vi "WCA_init.vi"(8 "Cartridge band":u32=10 max=10 step=1, 10 "Node address":u16=19 format="%.0x", 11 "CAN Interface":string="CAN0") -> (0 "error out 2":errorcluster {"code" format="%.0x"}, 1 "Detected CAN Nodes.":string, 2 "Slave Node in":cluster{"Address":i16, "Serial Number":i8[]} {"Serial Number" format="%.0x"; "Address" format="%.0x"}, 3 "ObjHandle out":u32, 4 "CAN nodes found on bus.":cluster{"Address":i8, "Serial Number":i8[]}[](array[cluster]) {"Serial Number" format="%.0x"; "Address" format="%.0x"})   [LabVIEW 2017]
uses:
  WCA_Global.vi
panel:
  out "Node index Bias":i32=-1
  # "Node Address"
  # "Serial Number"
  # "Node Address"
  # "Serial Number"
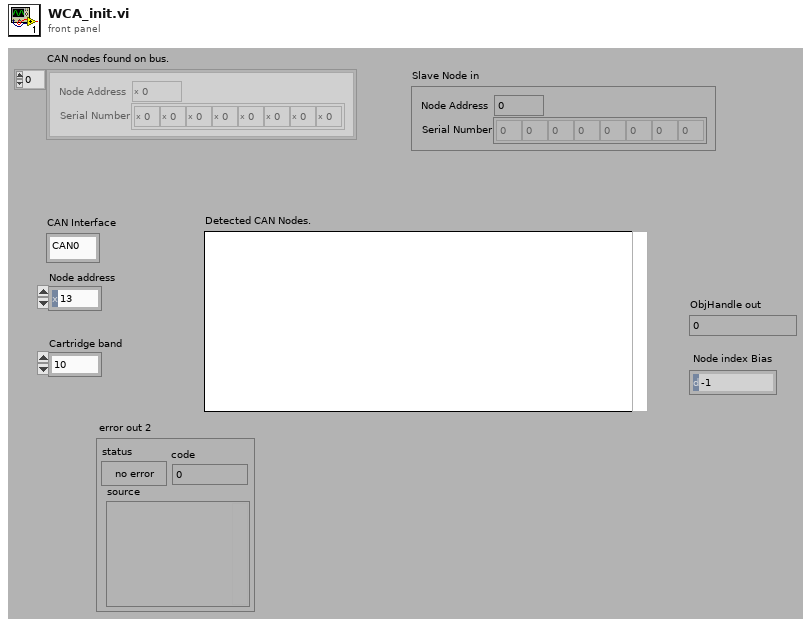
[diagram p1: front panel]
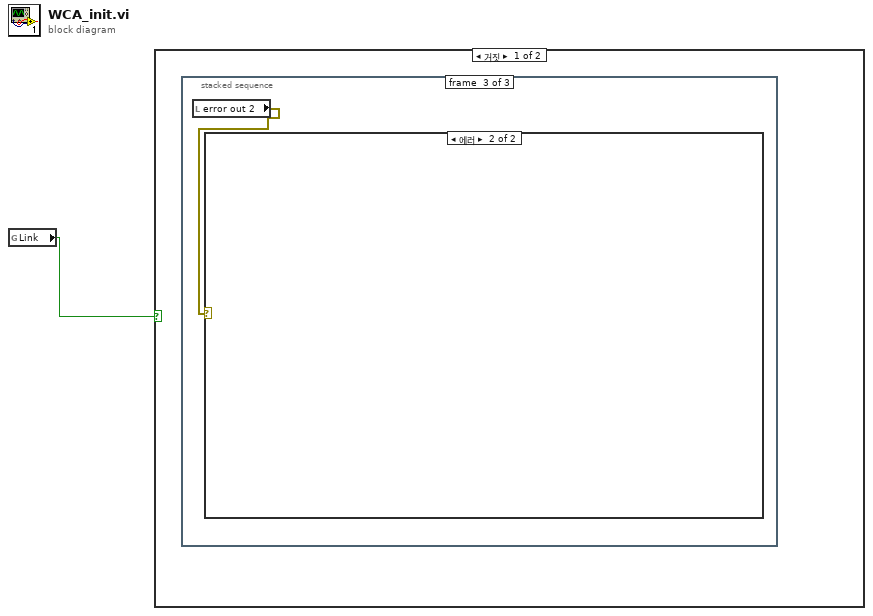
[diagram p0: block diagram]
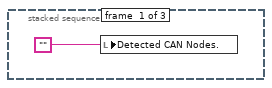
[diagram p2: hidden frame]
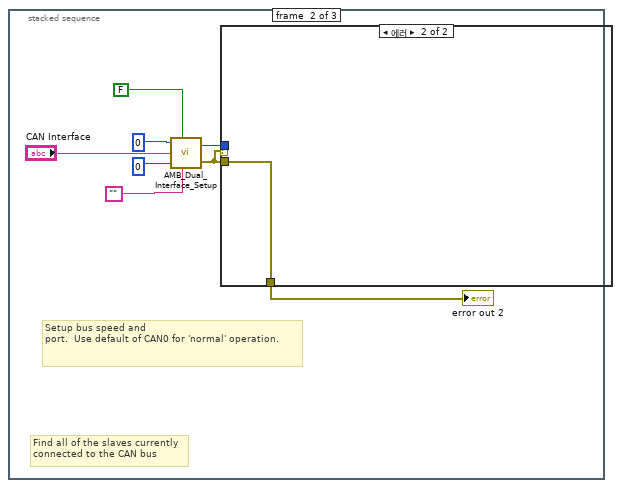
[diagram p3: hidden frame]
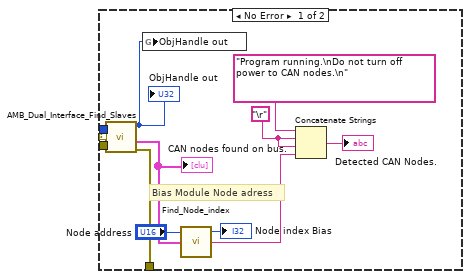
[diagram p4: hidden frame]
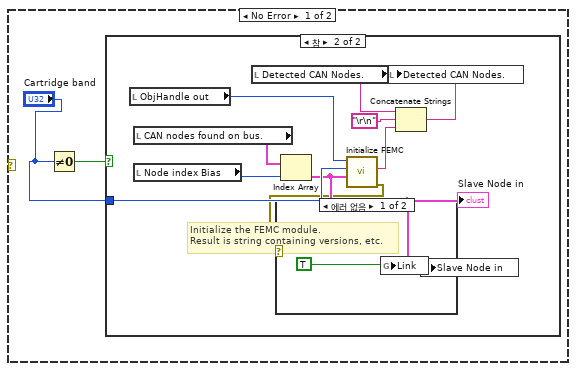
[diagram p5: hidden frame]
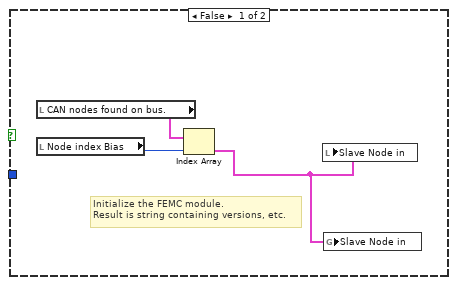
[diagram p6: hidden frame]
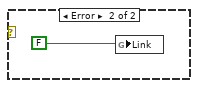
[diagram p7: hidden frame]
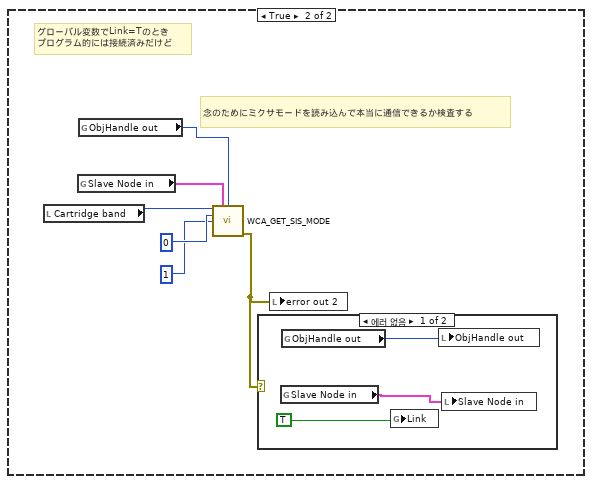
[diagram p8: hidden frame]
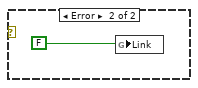
[diagram p9: hidden frame]
diagram:
  n1 = global read "WCA_Global.vi" "Link"() -> (w1:bool)
  n2 = case shown="거짓" w1 {
    frame False {
      n3 = stacked-sequence {
        frame #0 {
          n4 = local write "Detected CAN Nodes."("") -> ()
        }
        frame #1 {
          # "Find all of the slaves currently\nconnected to the CAN bus"
          # "Setup bus speed and\nport.  Use default of CAN0 for 'normal' operation."
          n5 = call "AMB_Dual_Interface_Setup.vi"("ABM"=i16 0, "TCP"=FALSE, "CAN Port In"="CAN Interface", "Port#"=u16 0, "Host"="") -> ("CAN Network\nObject \nHandle Out"=w10:u32, "error out"=w4:errorcluster)
          n6 = case shown="에러" w4 {
            tunnel: w10 -> [w21 _]
            tunnel: w4 -> [w20 w22]
            tunnel: [w11 w22] -> w3
            frame No Error {
              w15 = "\r"
              # "Bias Module Node adress"
              n7 = call "AMB_Dual_Interface_Find_Slaves.vi"("ObjHandle in"=w21, "error in"=w20) -> ("ObjHandle out"=w12:u32, "Node Array out"=w14:cluster{"Address":u16, "Serial Number":i8[]}[], "error out"=w11:errorcluster)  [unwired: 1 out]
              "ObjHandle out" <- w12
              "CAN nodes found on bus." <- w14
              n8 = global write "WCA_Global.vi" "ObjHandle out"(w12) -> ()
              n9 = call "Find_Node_index.vi"("Node Array out"=w14, "Node adress"="Node address") -> ("Message"=w19:string, "Node index"=→"Node index Bias":i32)  [unwired: 1 in, 1 out]
              n10 = Concatenate Strings("Program running.\nDo not turn off power to CAN nodes.\n", w15, w15, w19) -> (→"Detected CAN Nodes.":string)
            }
            frame Error {
            }
          }
          "error out 2" <- w3
        }
        frame #2 {
          n11 = local read "error out 2"() -> (w23:errorcluster)
          n12 = case shown="에러" w23 {
            frame No Error {
              n13 = Not Equal To 0?(x="Cartridge band") -> (x != 0?=w25:bool)
              n14 = case shown="참" w25 {
                tunnel: "Cartridge band" -> [_ w31]
                frame False {
                  # "Initialize the FEMC module.\nResult is string containing versions, etc."
                  n15 = local read "CAN nodes found on bus."() -> (w28:cluster{"Address":i8, "Serial Number":i8[]}[])
                  n16 = local read "Node index Bias"() -> (w27:i32)
                  n17 = Index Array(array=w28, index=w27) -> (element=w26:cluster{"Address":i8, "Serial Number":i8[]})
                  n18 = local write "Slave Node in"(w26) -> ()
                  n19 = global write "WCA_Global.vi" "Slave Node in"(w26) -> ()
                }
                frame True {
                  # "Initialize the FEMC module.\nResult is string containing versions, etc."
                  n20 = local read "ObjHandle out"() -> (w36:u32)
                  n21 = local read "CAN nodes found on bus."() -> (w38:cluster{"Address":i8, "Serial Number":i8[]}[])
                  n22 = local read "Node index Bias"() -> (w37:i32)
                  n23 = local read "Detected CAN Nodes."() -> (w35:string)
                  n24 = Index Array(array=w38, index=w37) -> (element=w30:cluster{"Address":i8, "Serial Number":i8[]})
                  "Slave Node in" <- w30
                  n25 = call "Initialize FEMC.vi"("Slave Node in"=w30, "Cartridge band"=w31, "ObjHandle in"=w36) -> ("error out"=w29:errorcluster, "Info String"=w33:string)  [unwired: 7 in]
                  n26 = case shown="에러 없음" w29 {
                    frame No Error {
                      n27 = global write "WCA_Global.vi" "Link"(TRUE) -> ()
                    }
                    frame Error {
                      n28 = global write "WCA_Global.vi" "Link"(FALSE) -> ()
                    }
                  }
                  n29 = Concatenate Strings(w35, "\r\n", w33) -> (w34:string)
                  n30 = local write "Detected CAN Nodes."(w34) -> ()
                  n31 = global write "WCA_Global.vi" "Slave Node in"(w30) -> ()
                }
              }
            }
            frame Error {
            }
          }
        }
      }
    }
    frame True {
      # "念のためにミクサモードを読み込んで本当に通信できるか検査する"
      # "グローバル変数でLink=Tのとき\nプログラム的には接続済みだけど"
      n32 = local read "Cartridge band"() -> (w44:u32)
      n33 = global read "WCA_Global.vi" "Slave Node in"() -> (w45:cluster{"Address":i16, "Serial Number":i8[]})
      n34 = global read "WCA_Global.vi" "ObjHandle out"() -> (w46:u32)
      n35 = call "WCA_GET_SIS_MODE.vi"("Cartridge Band"=w44, "Slave Node in"=w45, "ObjHandle in"=w46, "POL"=0, "sb"=1) -> ("error out"=w41:errorcluster)  [unwired: 8 in, 2 out]
      n36 = case shown="에러 없음" w41 {
        frame No Error {
          n37 = global read "WCA_Global.vi" "Slave Node in"() -> (w48:cluster{"Address":i16, "Serial Number":i8[]})
          n38 = global read "WCA_Global.vi" "ObjHandle out"() -> (w47:u32)
          n39 = global write "WCA_Global.vi" "Link"(TRUE) -> ()
          n40 = local write "ObjHandle out"(w47) -> ()
          n41 = local write "Slave Node in"(w48) -> ()
        }
        frame Error {
          n42 = global write "WCA_Global.vi" "Link"(FALSE) -> ()
        }
      }
      n43 = local write "error out 2"(w41) -> ()
    }
  }
